vi "Finish.vi"(4 "error in":errorcluster) -> ()   [LabVIEW 2013]
doc: "This VI is called just before exiting. It is expected to close I/O refnum, save collected data, etc."
uses:
  <vilib>/Rock Robotics/WPI/Solenoid/WPI_SolenoidValue.ctl
  <vilib>/Rock Robotics/WPI/RobotDrive/WPI_RobotDriveGetSetRefNum.vi
  <vilib>/Rock Robotics/WPI/Joystick/WPI_JoystickGetSetRefNum.vi
  <vilib>/Rock Robotics/WPI/Solenoid/WPI_SolenoidSetEnum.vi
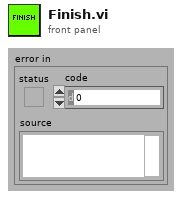
[diagram p1: front panel]
types:
  T1 = typedef "WPI_DigitalInputDevRef.ctl" = cluster{"DevStatus":errorcluster, "DIO Channel":T2, "Digital Module":T3}
  T2 = typedef "FPGA_DIOChannel.ctl" = enum8{"DIO 1", "DIO 2", "DIO 3", "DIO 4", "DIO 5", "DIO 6", "DIO 7", "DIO 8", "DIO 9", "DIO 10", "DIO 11", "DIO 12", "DIO 13", "DIO 14", "Invalid"}
  T3 = typedef "FPGA_TypedefDigitalModule.ctl" = enum16{"Digital Module 1", "Digital Module 2"}
  T4 = typedef "WPI_JoystickDevRef.ctl" = cluster{"Device":T5}
  T5 = typedef "WPI_JoystickDeviceEnum.ctl" = enum16{"USB 1", "USB 2", "USB 3", "USB 4", "Kinect 1", "Kinect 2"}
  T6 = typedef "WPI_CameraDevRef.ctl" = cluster{"Camera Address":string, "CameraStatus":errorcluster, "Acquire Image Notifier":refnum<notifier>}
  T7 = typedef "WPI_RobotDriveDevRef.ctl" = cluster{"DevStatus":errorcluster, "Motors[]":T8[], "Square Inputs":bool, "Max Output":dbl, "Isochronous":bool}
  T8 = typedef "WPI_MotorControlDeviceRef.ctl" = cluster{"DeviceStatus":errorcluster, "Type":enum16{"PWM", "CAN"}, "PWM":cluster{"Digital Module":T3, "PWM Channel":T9, "DeadBand":T10}, "CAN":cluster{"Device Number":u8, "Control Mode":T11, "Semaphore":T12, "Max Vout":dbl}, "Invert":bool, "TransformRef":T13, "InvTransformRef":T13}
  T9 = typedef "FPGA_DIOPWMChannel.ctl" = enum8{"PWM 1", "PWM 2", "PWM 3", "PWM 4", "PWM 5", "PWM 6", "PWM 7", "PWM 8", "PWM 9", "PWM 10", "Invalid"}
  T10 = typedef "WPI_PWMDeadband.ctl" = cluster{"Name":string, "maxPositivePwm":i32, "minPositivePwm":i32, "centerPwm":i32, "maxNegativePwm":i32, "minNegativePwm":i32, "angularRange":u16}
  T11 = typedef "WPI_CANJaguar_ControlMode.ctl" = enum8{"Percent VBus", "Current", "Speed", "Position", "Voltage"}
  T12 = typedef "Semaphore RefNum" = refnum<k1>
  T13 = typedef "WPI_PWMTransform_ConPane.ctl" = refnum<vi>
  T14 = typedef "WPI_EncoderDevRef.ctl" = cluster{"DevStatus":errorcluster, "EncoderIndex":T15, "CounterIndex":T16, "DistancePerCount":dbl, "Decoding Type":T17}
  T15 = typedef "FPGA_EncoderIdx.ctl" = enum8{"Enc 0", "Enc 1", "Enc 2", "Enc 3", "Invalid"}
  T16 = typedef "FPGA_CounterCtrSystemIndex.ctl" = enum8{"Ctr 0", "Ctr 1", "Ctr 2", "Ctr 3", "Ctr 4", "Ctr 5", "Ctr 6", "Ctr 7", "Invalid"}
  T17 = typedef "WPI_EncoderType.ctl" = enum16{"1x", "2x", "4x"}
  T18 = typedef "WPI_SolenoidDevRef.ctl" = cluster{"DevStatus":errorcluster, "Solenoid Module":T19, "Forward Solenoid Channel":T20, "Reverse Solenoid Channel":T20}
  T19 = typedef "FPGA_TypedefSolenoidModule.ctl" = enum16{"Solenoid Module 1", "Solenoid Module 2"}
  T20 = typedef "WPI_SolenoidChannel.ctl" = enum8{"Solenoid 1", "Solenoid 2", "Solenoid 3", "Solenoid 4", "Solenoid 5", "Solenoid 6", "Solenoid 7", "Solenoid 8", "Invalid"}
  T21 = typedef "WPI_SolenoidValue.ctl" = enum16{"Off", "On", "Forward", "Reverse"}
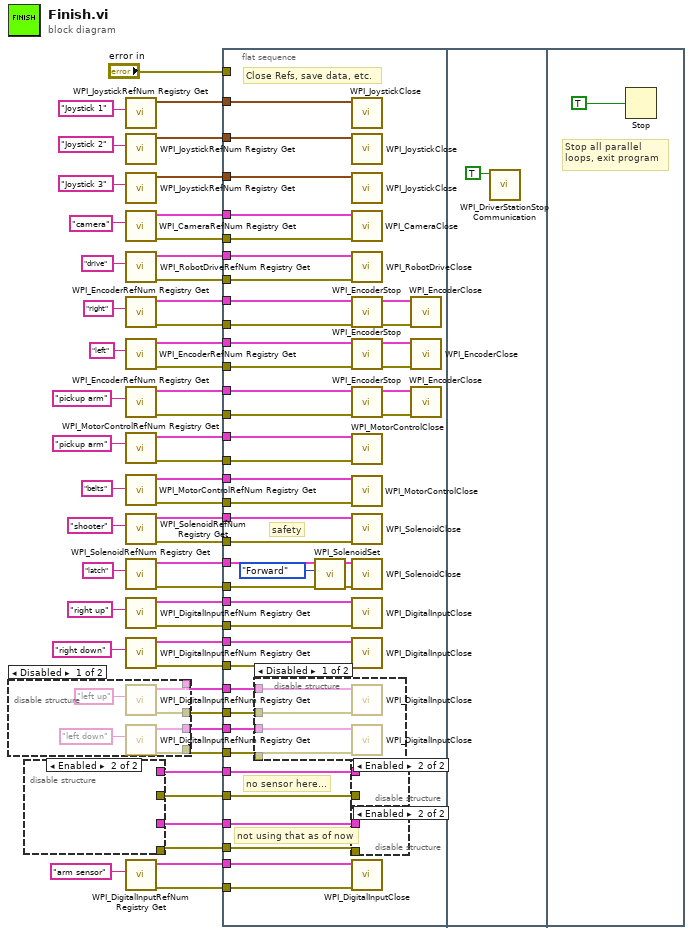
[diagram p0: block diagram]
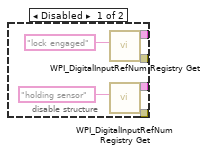
[diagram p3: hidden frame]
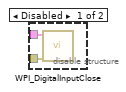
[diagram p5: hidden frame]
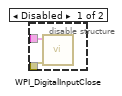
[diagram p6: hidden frame]
diagram:
  n1 = disable-structure shown="Disabled" {
    disable-tunnel: [w55 _] -> w11
    disable-tunnel: [w54 _] -> w10
    disable-tunnel: [w53 _] -> w9
    disable-tunnel: [w52 _] -> w8
    frame Disabled {
      n2 = call <vilib>:"WPI_DigitalInputRefNum Registry Get.vi"("refnum name"="left up") -> ("error out"=w54:errorcluster, "DigitalInputDevRef"=w55:T1)  [unwired: 9 in]
      n3 = call <vilib>:"WPI_DigitalInputRefNum Registry Get.vi"("refnum name"="left down") -> ("error out"=w52:errorcluster, "DigitalInputDevRef"=w53:T1)  [unwired: 9 in]
    }
    frame Enabled {
    }
  }
  n4 = disable-structure shown="Enabled" {
    disable-tunnel: [w63 _] -> w5
    disable-tunnel: [w62 _] -> w4
    disable-tunnel: [w60 _] -> w2
    disable-tunnel: [w59 _] -> w1
    frame Disabled {
      n5 = call <vilib>:"WPI_DigitalInputRefNum Registry Get.vi"("refnum name"="lock engaged") -> ("error out"=w60:errorcluster, "DigitalInputDevRef"=w59:T1)  [unwired: 9 in]
      n6 = call <vilib>:"WPI_DigitalInputRefNum Registry Get.vi"("refnum name"="holding sensor") -> ("error out"=w63:errorcluster, "DigitalInputDevRef"=w62:T1)  [unwired: 9 in]
    }
    frame Enabled {
    }
  }
  n7 = call <vilib>:"WPI_JoystickRefNum Registry Get.vi"("refnum name"="Joystick 1") -> ("JoystickDevRef"=w50:T4)  [unwired: 1 in, 9 out]
  n8 = call <vilib>:"WPI_JoystickRefNum Registry Get.vi"("refnum name"="Joystick 2") -> ("JoystickDevRef"=w47:T4)  [unwired: 1 in, 9 out]
  n9 = call <vilib>:"WPI_JoystickRefNum Registry Get.vi"("refnum name"="Joystick 3") -> ("JoystickDevRef"=w44:T4)  [unwired: 1 in, 9 out]
  n10 = call <vilib>:"WPI_CameraRefNum Registry Get.vi"("refnum name"="camera") -> ("error out"=w37:errorcluster, "CameraDevRef"=w49:T6)  [unwired: 1 in, 8 out]
  n11 = call <vilib>:"WPI_RobotDriveRefNum Registry Get.vi"("refnum name"="drive") -> ("error out"=w36:errorcluster, "RobotDriveDevRef"=w42:T7)  [unwired: 9 in]
  n12 = call <vilib>:"WPI_EncoderRefNum Registry Get.vi"("refnum name"="right") -> ("error out"=w35:errorcluster, "EncoderDevRef"=w39:T14)  [unwired: 9 in]
  n13 = call <vilib>:"WPI_EncoderRefNum Registry Get.vi"("refnum name"="left") -> ("error out"=w34:errorcluster, "EncoderDevRef"=w38:T14)  [unwired: 9 in]
  n14 = call <vilib>:"WPI_EncoderRefNum Registry Get.vi"("refnum name"="pickup arm") -> ("error out"=w33:errorcluster, "EncoderDevRef"=w31:T14)  [unwired: 9 in]
  n15 = call <vilib>:"WPI_MotorControlRefNum Registry Get.vi"("refnum name"="pickup arm") -> ("error out"=w27:errorcluster, "MotorControlDevRef"=w28:T8)  [unwired: 9 in]
  n16 = call <vilib>:"WPI_MotorControlRefNum Registry Get.vi"("refnum name"="belts") -> ("error out"=w25:errorcluster, "MotorControlDevRef"=w26:T8)  [unwired: 9 in]
  n17 = call <vilib>:"WPI_SolenoidRefNum Registry Get.vi"("refnum name"="shooter") -> ("error out"=w23:errorcluster, "SolenoidDevRef"=w24:T18)  [unwired: 9 in]
  n18 = call <vilib>:"WPI_SolenoidRefNum Registry Get.vi"("refnum name"="latch") -> ("error out"=w19:errorcluster, "SolenoidDevRef"=w20:T18)  [unwired: 9 in]
  n19 = call <vilib>:"WPI_DigitalInputRefNum Registry Get.vi"("refnum name"="right up") -> ("error out"=w14:errorcluster, "DigitalInputDevRef"=w15:T1)  [unwired: 9 in]
  n20 = call <vilib>:"WPI_DigitalInputRefNum Registry Get.vi"("refnum name"="right down") -> ("error out"=w12:errorcluster, "DigitalInputDevRef"=w13:T1)  [unwired: 9 in]
  n21 = call <vilib>:"WPI_DigitalInputRefNum Registry Get.vi"("refnum name"="arm sensor") -> ("error out"=w7:errorcluster, "DigitalInputDevRef"=w6:T1)  [unwired: 9 in]
  n22 = flat-sequence {
    tunnel: w50 -> [w107]
    tunnel: w49 -> [w106]
    tunnel: w47 -> [w105]
    tunnel: w44 -> [w104]
    tunnel: w42 -> [w103]
    tunnel: w39 -> [w102]
    tunnel: w38 -> [w95]
    tunnel: w37 -> [w99]
    tunnel: w36 -> [w98]
    tunnel: w35 -> [w97]
    tunnel: w34 -> [w96]
    tunnel: w33 -> [w91]
    tunnel: w31 -> [w90]
    tunnel: w28 -> [w88]
    tunnel: w27 -> [w87]
    tunnel: w26 -> [w85]
    tunnel: w25 -> [w86]
    tunnel: w24 -> [w83]
    tunnel: w23 -> [w84]
    tunnel: w20 -> [w67]
    tunnel: w19 -> [w65]
    tunnel: "error in" -> [_]
    tunnel: w15 -> [w78]
    tunnel: w14 -> [w79]
    tunnel: w13 -> [w77]
    tunnel: w12 -> [w80]
    tunnel: w11 -> [w76]
    tunnel: w10 -> [w81]
    tunnel: w9 -> [w75]
    tunnel: w8 -> [w82]
    tunnel: w4 -> [w73]
    tunnel: w5 -> [w72]
    tunnel: w6 -> [w74]
    tunnel: w7 -> [w71]
    tunnel: w1 -> [w70]
    tunnel: w2 -> [w69]
    frame #0 {
      # "safety"
      # "no sensor here..."
      # "not using that as of now"
      # "Close Refs, save data, etc."
      n23 = disable-structure shown="Disabled" {
        disable-tunnel: w82 -> [w111 _]
        disable-tunnel: w81 -> [w110 _]
        disable-tunnel: w76 -> [w109 _]
        disable-tunnel: w75 -> [w108 _]
        frame Disabled {
          n24 = call <vilib>:"WPI_DigitalInputClose.vi"("error in (no error)"=w110, "DigitalInputDevRef"=w109) -> ()  [unwired: 9 in, 1 out]
          n25 = call <vilib>:"WPI_DigitalInputClose.vi"("error in (no error)"=w111, "DigitalInputDevRef"=w108) -> ()  [unwired: 9 in, 1 out]
        }
        frame Enabled {
        }
      }
      n26 = call-poly <vilib>:"WPI_SolenoidSet.vi"("error in (no error)"=w65, "Value"=WPI_SolenoidValue."Forward", "SolenoidDevRef"=w67) -> ("error out"=w66:errorcluster, "SolenoidDevRef"=w68:T18)  [unwired: 7 in]
      n27 = call <vilib>:"WPI_JoystickClose.vi"("JoystickDevRef"=w107) -> ()  [unwired: 11 out]
      n28 = call <vilib>:"WPI_JoystickClose.vi"("JoystickDevRef"=w105) -> ()  [unwired: 11 out]
      n29 = call <vilib>:"WPI_JoystickClose.vi"("JoystickDevRef"=w104) -> ()  [unwired: 11 out]
      n30 = call <vilib>:"WPI_CameraClose.vi"("error in (no error)"=w99, "CameraDevRef"=w106) -> ()  [unwired: 10 out]
      n31 = call <vilib>:"WPI_RobotDriveClose.vi"("error in (no error)"=w98, "RobotDriveDevRef"=w103) -> ()  [unwired: 9 in, 1 out]
      n32 = call <vilib>:"WPI_EncoderStop.vi"("error in (no error)"=w97, "EncoderDevRef"=w102) -> ("error out"=w101:errorcluster, "EncoderDevRef"=w100:T14)  [unwired: 8 in]
      n33 = call <vilib>:"WPI_EncoderStop.vi"("error in (no error)"=w96, "EncoderDevRef"=w95) -> ("error out"=w93:errorcluster, "EncoderDevRef"=w94:T14)  [unwired: 8 in]
      n34 = call <vilib>:"WPI_EncoderStop.vi"("error in (no error)"=w91, "EncoderDevRef"=w90) -> ("error out"=w92:errorcluster, "EncoderDevRef"=w89:T14)  [unwired: 8 in]
      n35 = call <vilib>:"WPI_MotorControlClose.vi"("error in (no error)"=w87, "MotorControlDevRef"=w88) -> ()  [unwired: 9 in, 1 out]
      n36 = call <vilib>:"WPI_MotorControlClose.vi"("error in (no error)"=w86, "MotorControlDevRef"=w85) -> ()  [unwired: 9 in, 1 out]
      n37 = call <vilib>:"WPI_SolenoidClose.vi"("error in (no error)"=w84, "SolenoidDevRef"=w83) -> ()  [unwired: 9 in, 1 out]
      n38 = call <vilib>:"WPI_SolenoidClose.vi"("error in (no error)"=w66, "SolenoidDevRef"=w68) -> ()  [unwired: 9 in, 1 out]
      n39 = call <vilib>:"WPI_DigitalInputClose.vi"("error in (no error)"=w79, "DigitalInputDevRef"=w78) -> ()  [unwired: 9 in, 1 out]
      n40 = call <vilib>:"WPI_DigitalInputClose.vi"("error in (no error)"=w80, "DigitalInputDevRef"=w77) -> ()  [unwired: 9 in, 1 out]
      n41 = disable-structure shown="Enabled" {
        disable-tunnel: w70 -> [w113 _]
        disable-tunnel: w69 -> [w112 _]
        frame Disabled {
          n42 = call <vilib>:"WPI_DigitalInputClose.vi"("error in (no error)"=w112, "DigitalInputDevRef"=w113) -> ()  [unwired: 9 in, 1 out]
        }
        frame Enabled {
        }
      }
      n43 = disable-structure shown="Enabled" {
        disable-tunnel: w73 -> [w115 _]
        disable-tunnel: w72 -> [w114 _]
        frame Disabled {
          n44 = call <vilib>:"WPI_DigitalInputClose.vi"("error in (no error)"=w114, "DigitalInputDevRef"=w115) -> ()  [unwired: 9 in, 1 out]
        }
        frame Enabled {
        }
      }
      n45 = call <vilib>:"WPI_DigitalInputClose.vi"("error in (no error)"=w71, "DigitalInputDevRef"=w74) -> ()  [unwired: 9 in, 1 out]
      n46 = call <vilib>:"WPI_EncoderClose.vi"("error in (no error)"=w101, "EncoderDevRef"=w100) -> ()  [unwired: 9 in, 1 out]
      n47 = call <vilib>:"WPI_EncoderClose.vi"("error in (no error)"=w93, "EncoderDevRef"=w94) -> ()  [unwired: 9 in, 1 out]
      n48 = call <vilib>:"WPI_EncoderClose.vi"("error in (no error)"=w92, "EncoderDevRef"=w89) -> ()  [unwired: 9 in, 1 out]
    }
    frame #1 {
      n49 = call <vilib>:"WPI_DriverStationStop Communication.vi"("StopCommunication"=TRUE) -> ()  [unwired: 10 in, 1 out]
    }
    frame #2 {
      # "Stop all parallel\nloops, exit program"
      n50 = Stop(stop? (T)=TRUE ("Quit")) -> ()
    }
  }
